vi "Remove Created Queue.vi"(9 "Self Queue Alias":string, 10 "Queue Mailbox in":refnum<data-value>) -> (0 "error out":errorcluster, 2 "Queue Mailbox out":refnum<data-value>)   [LabVIEW 2021, in "jettl.lvlib" / "Addresses.lvlib"]
uses:
  Addresses.lvlib
  Addresses/Addresses.lvclass
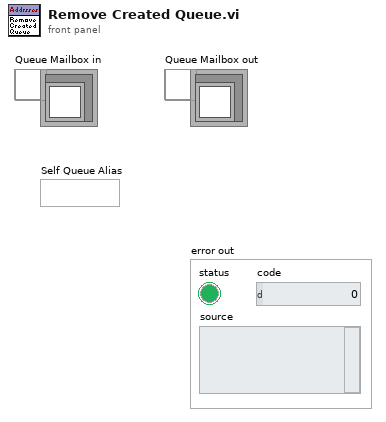
[diagram p1: front panel]
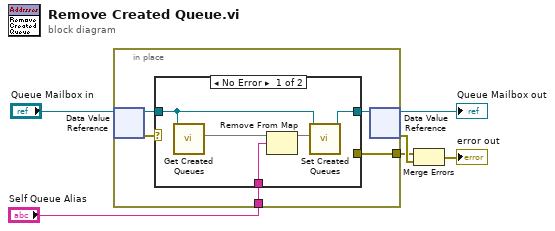
[diagram p0: block diagram]
diagram:
  n1 = in-place {
    in-place-border: [w11] -> w2
    in-place-border: "Self Queue Alias" -> [w8]
    n2 = in-place-dvr #1("Queue Mailbox in") -> (w9:refnum<class "Addresses.lvclass">, w10:errorcluster)
    n3 = case shown="No Error" w10 {
      selector: w10 -> [_ w18]
      tunnel: w9 -> [w13 w17]
      tunnel: [_ w18] -> w11
      tunnel: w8 -> [w15 _]
      tunnel: [w12 w17] -> w7
      frame No Error {
        n4 = call "Get Created Queues.vi"("Queue Mailbox in"=w13) -> ("Created Queues"=w16:map{string, refnum<data-value>})  [unwired: 10 in]
        n5 = Remove From Map(10:w15, 11:w16) -> (3:w14:map{string, refnum<data-value>})  [unwired: 2 out]
        n6 = call "Set Created Queues.vi"("Created Queues"=w14, "Queue Mailbox in"=w13) -> ("Queue Mailbox out"=w12:refnum<class "Addresses.lvclass">)  [unwired: 9 in]
      }
      frame Error {
      }
    }
    n7 = in-place-dvr #1(w7) -> (→"Queue Mailbox out":refnum<data-value>, w3:errorcluster)
  }
  n8 = Merge Errors(w2, w3) -> (→"error out":errorcluster)
